vi "laser_control of Tank 1.vi"(4 "error out":errorcluster, 5 "Boolean":bool, 7 "FPGA VI Reference Out":refnum<k20>) -> (0 "error out 2":errorcluster, 3 "FPGA VI Reference Out 2":refnum<k20>)   [LabVIEW 2012]
panel:
  in  "stop":bool
  in  "i":dbl
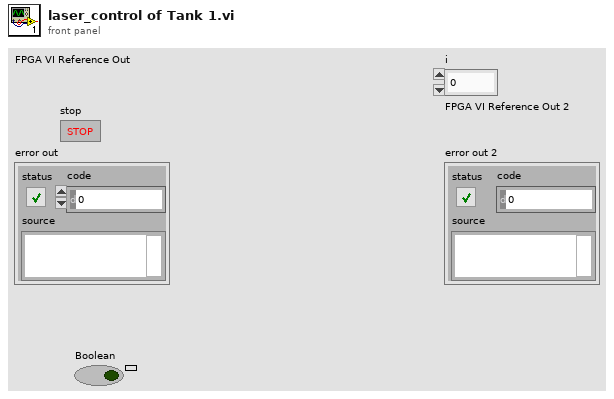
[diagram p1: front panel]
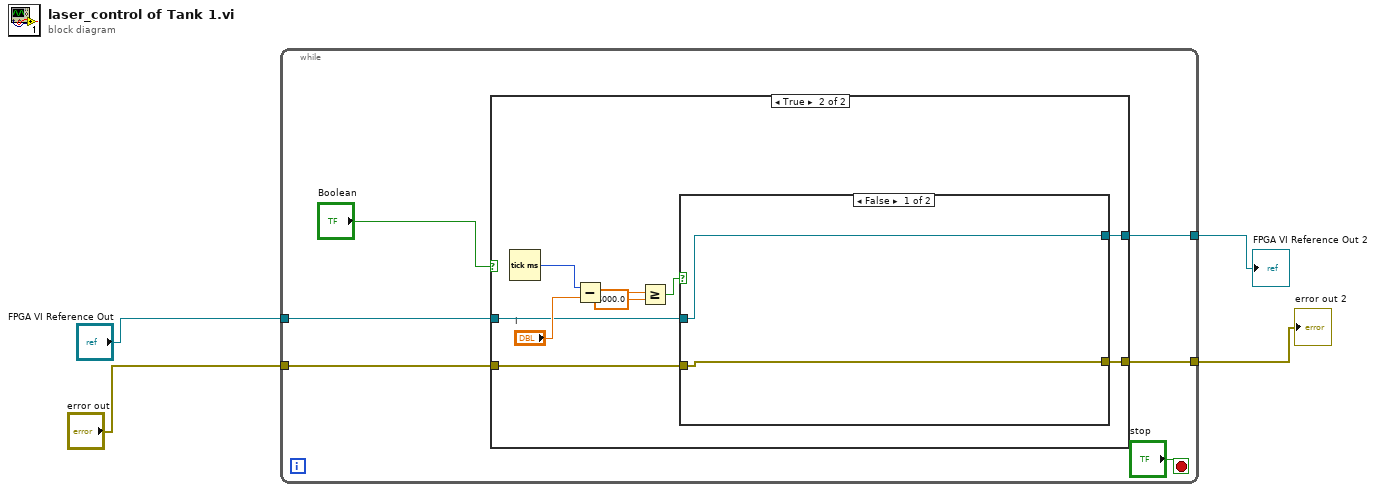
[diagram p0: block diagram]
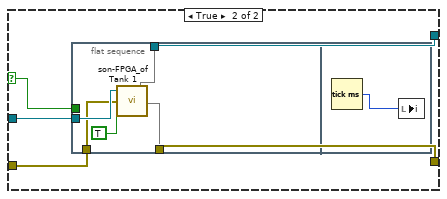
[diagram p3: hidden frame]
diagram:
  n1 = while {
    tunnel: "FPGA VI Reference Out" -> [w8]
    tunnel: "error out" -> [w7]
    tunnel: [w6] -> w2
    tunnel: [w5] -> w1
    stop <- "stop" stop-if-true
    n2 = case shown="True" "Boolean" {
      tunnel: w8 -> [w12 w16]
      tunnel: w7 -> [w11 w15]
      tunnel: [w12 w14] -> w6
      tunnel: [w11 w13] -> w5
      frame False {
      }
      frame True {
        n3 = Tick Count (ms)() -> (millisecond timer value=w18:u32)
        n4 = Subtract(x=w18, y="i") -> (x-y=w21:dbl)
        n5 = Greater Or Equal?(x=w21, y=6000.0) -> (x >= y?=w19:bool)
        n6 = case shown="False" w19 {
          selector: w19 -> [_ w28]
          tunnel: w16 -> [w23 w27]
          tunnel: w15 -> [w22 w26]
          tunnel: [w23 w25] -> w14
          tunnel: [w22 w24] -> w13
          frame False {
          }
          frame True {
            n7 = flat-sequence {
              tunnel: w28 -> [_]
              tunnel: w27 -> [w32]
              tunnel: w26 -> [w31]
              tunnel: [w30] -> w25
              tunnel: [w29] -> w24
              frame #0 {
                n8 = call "son-FPGA_of Tank 1.vi"("Port9/DIO8"=TRUE, "error out"=w31, "FPGA VI Reference Out"=w32) -> (0:w29, 2:w30)  [unwired: 1 in]
              }
              frame #1 {
                n9 = Tick Count (ms)() -> (millisecond timer value=w34:u32)
                n10 = local write "i"(w34) -> ()
              }
            }
          }
        }
      }
    }
  }
  "FPGA VI Reference Out 2" <- w2
  "error out 2" <- w1
